vi "Marshal.vi"(8 "error in (no error)":errorcluster, 11 "int32 in":refnum<class "fixed32.lvclass">) -> (0 "error out":errorcluster, 2 "Buffer":u8[](array[numeric]), 3 "int32 out":refnum<class "fixed32.lvclass">)   [LabVIEW 2020, in "Protobuf RAW.lvlib" / "fixed32.lvclass"]
uses:
  fixed32.lvclass
  fixed32.lvclass/fixed32.ctl
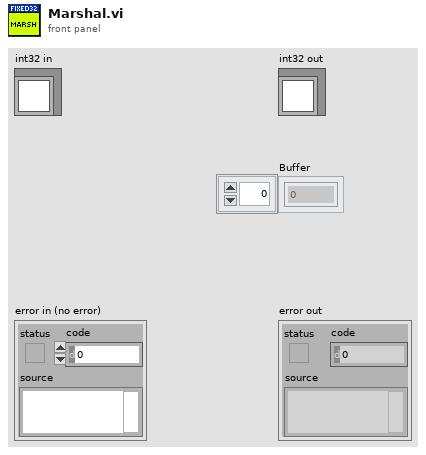
[diagram p1: front panel]
types:
  T1 = enum16{"big-endian, network order", "native, host order", "little-endian"}
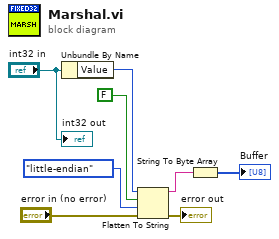
[diagram p0: block diagram]
diagram:
  n1 = Unbundle By Name("int32 in") -> ("Value"=w1:u32)
  n2 = Flatten To String(anything=w1, prepend array or string size? (T)=FALSE, byte order (0:big-endian, network order)=T1."little-endian", error in (no error)="error in (no error)") -> (data string=w5:string, error out=→"error out":errorcluster)  [unwired: 1 out]
  n3 = String To Byte Array(string=w5) -> (unsigned byte array=→"Buffer":u8[])
  "int32 out" <- "int32 in"
